vi "Transmit_Log_File_FGV.vi"(7 "Session name":string, 8 "error in (no error)":errorcluster, 9 "Command":enum16{"Initialize", "Update", "Stop"}(ring), 10 "Time (ms)":u32, 11 "Processed bytes":u8[](array[numeric])) -> (0 "error out":errorcluster, 3 "Receive Log File Path":path)   [LabVIEW 2017]
uses:
  <vilib>/Utility/file.llb/Write Delimited Spreadsheet (string).vi
  <vilib>/Utility/file.llb/Write Delimited Spreadsheet (I64).vi
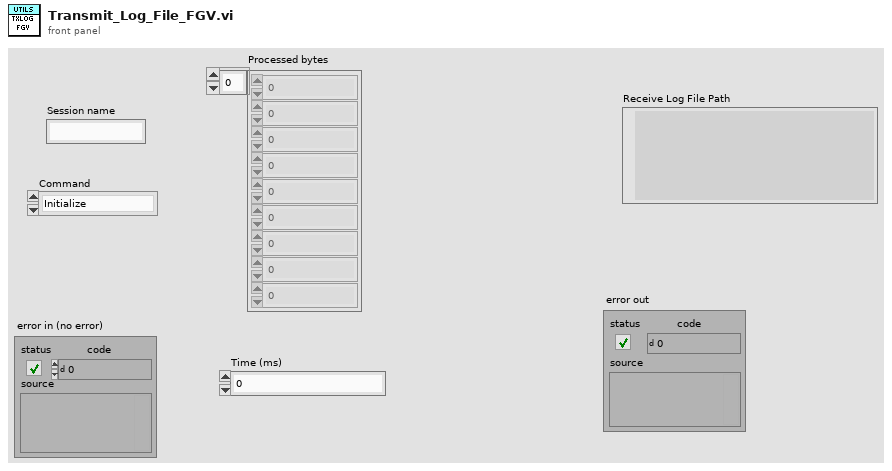
[diagram p1: front panel]
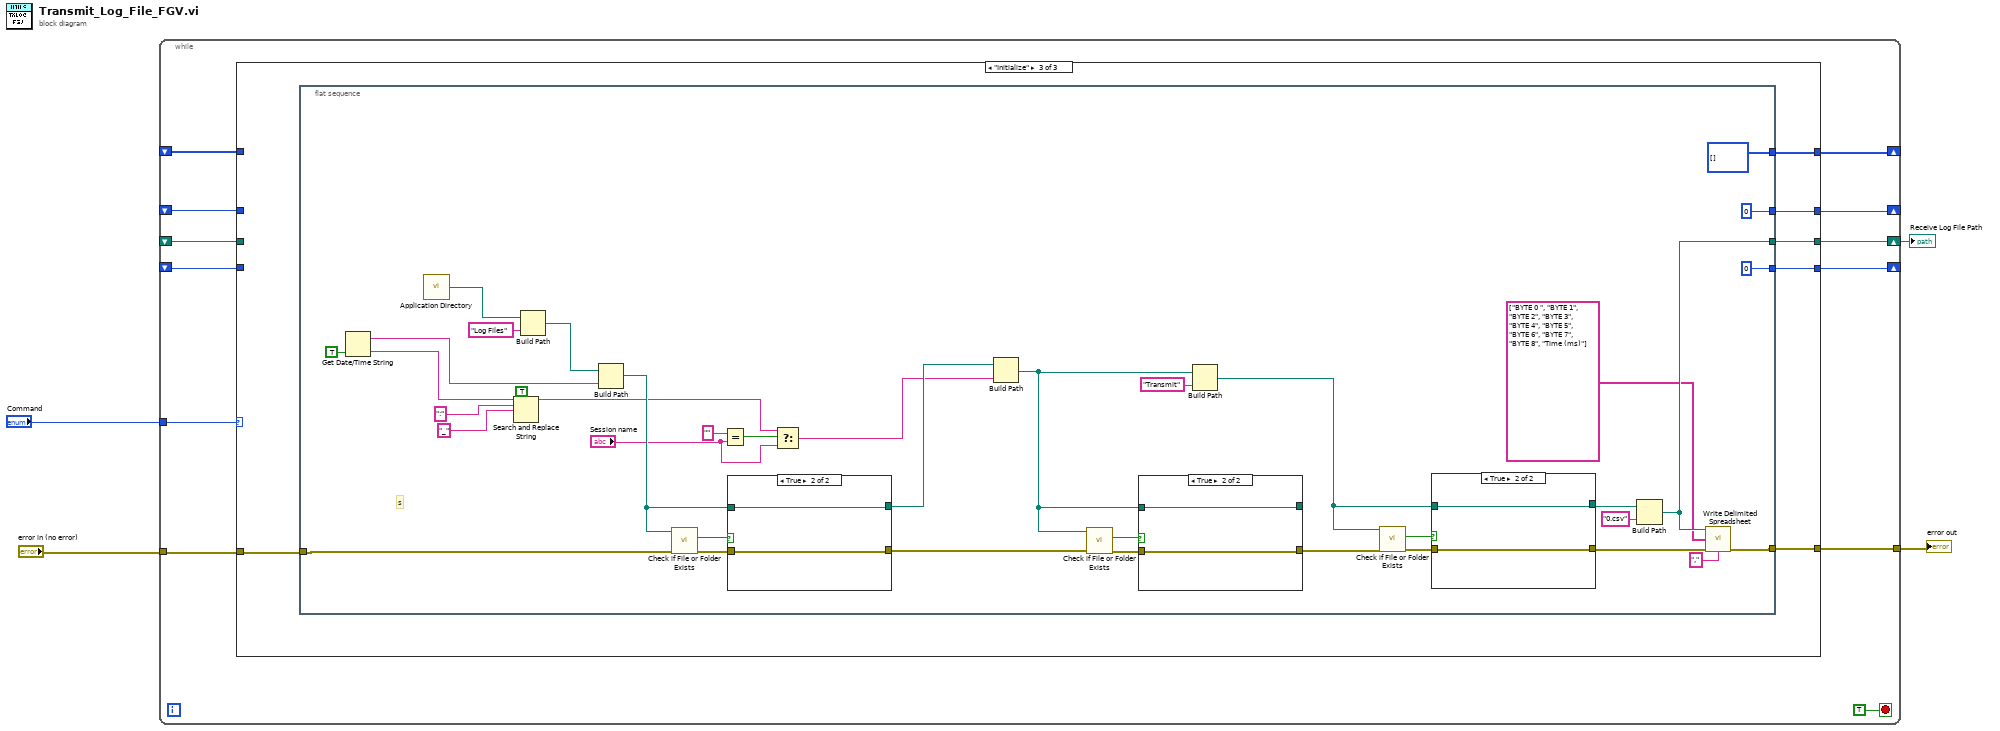
[diagram p0: block diagram]
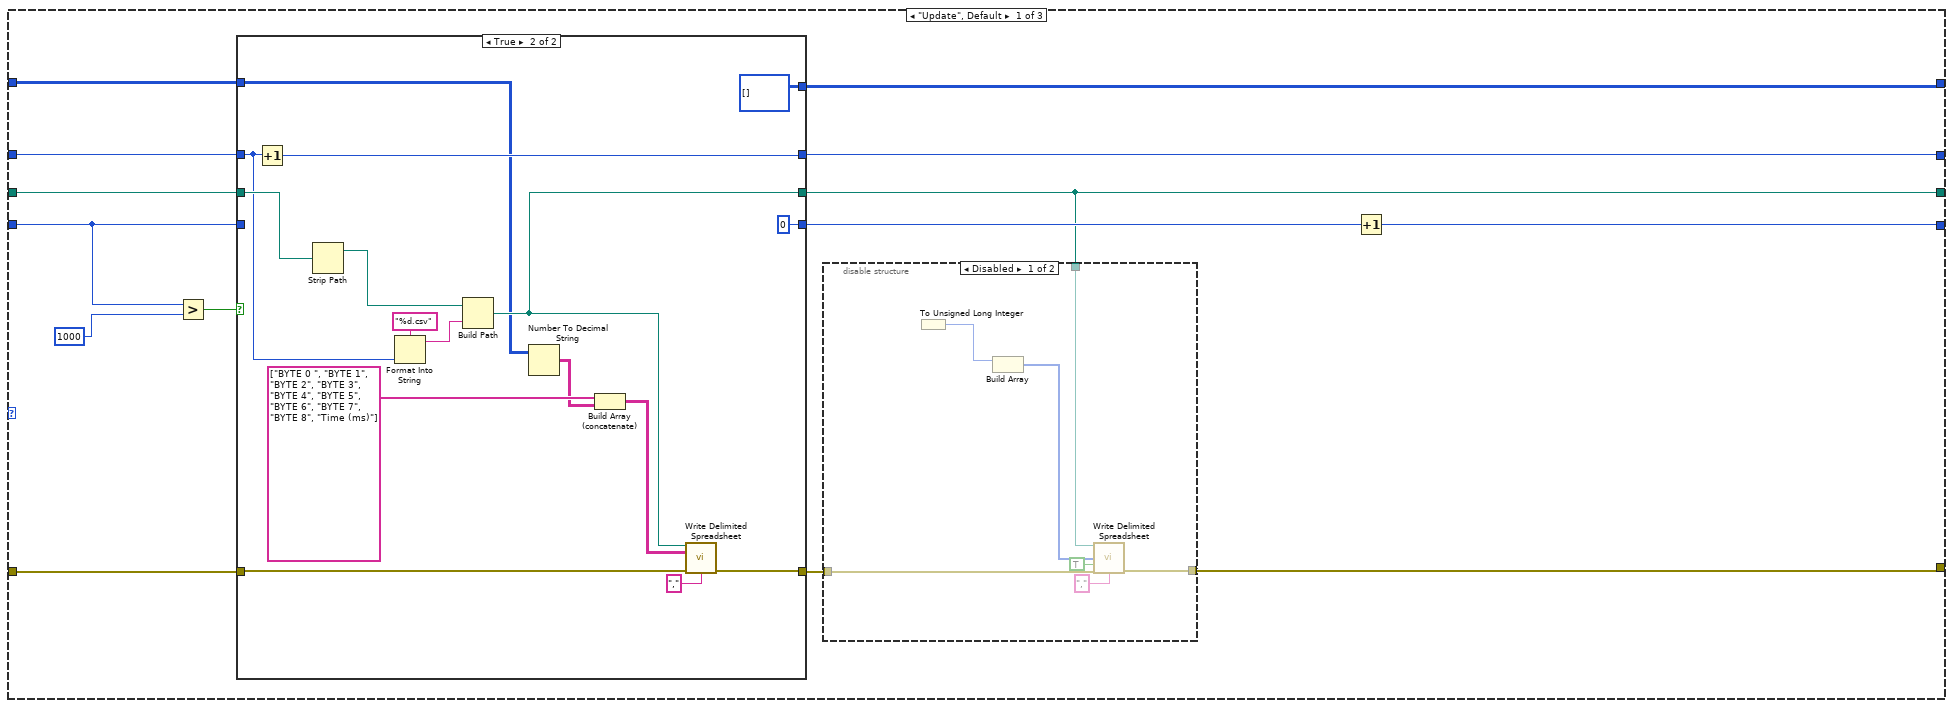
[diagram p2: hidden frame]
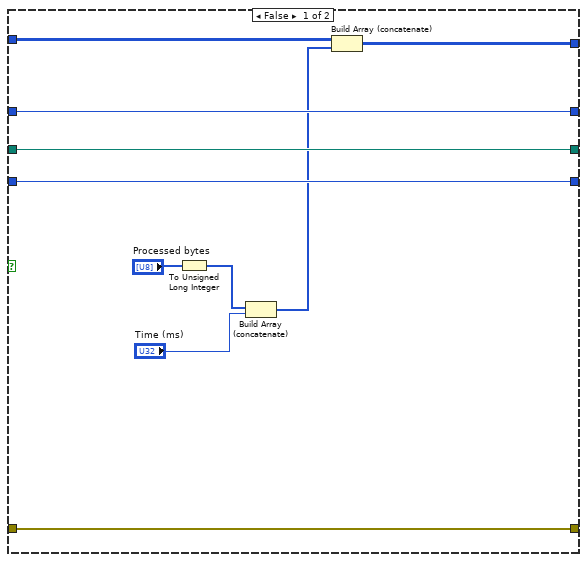
[diagram p4: hidden frame]
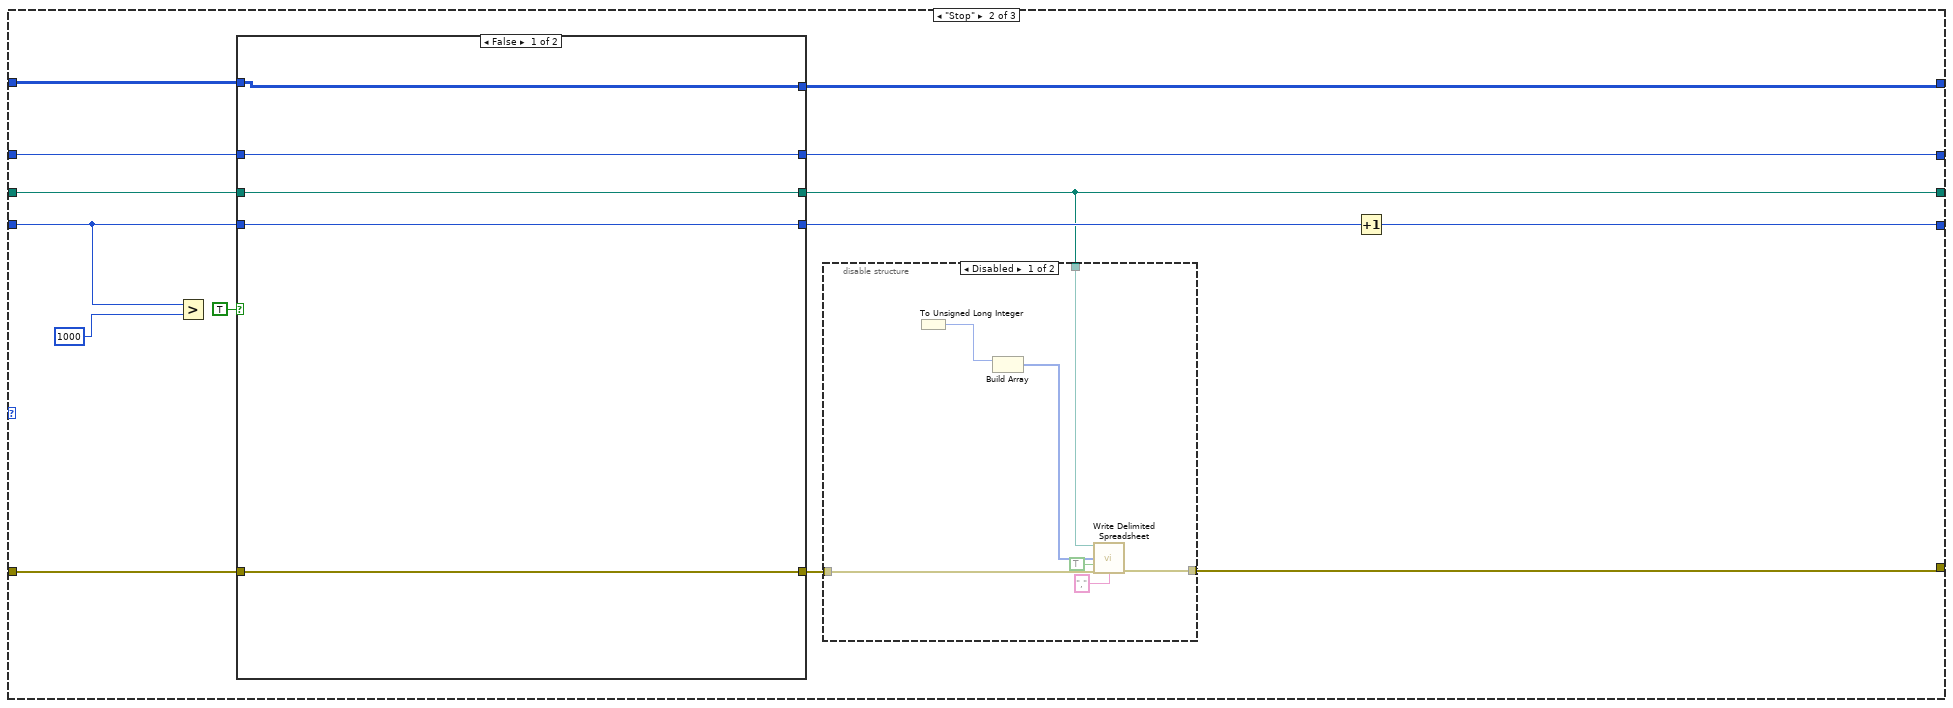
[diagram p5: hidden frame]
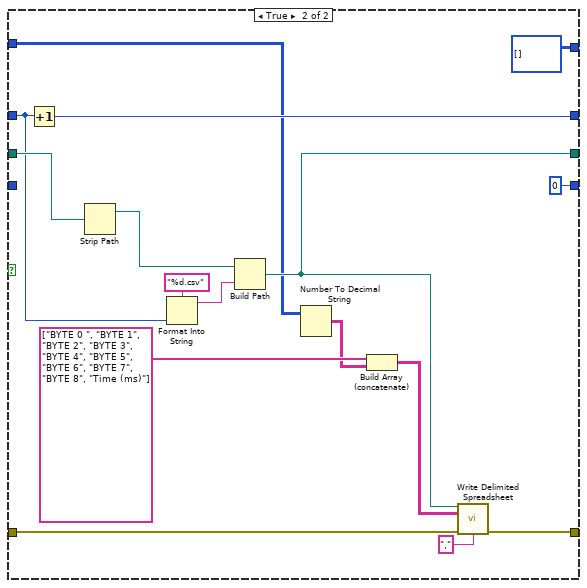
[diagram p7: hidden frame]
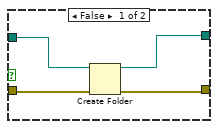
[diagram p8: hidden frame]
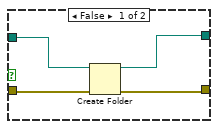
[diagram p9: hidden frame]
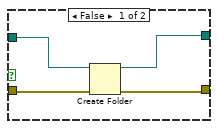
[diagram p10: hidden frame]
diagram:
  n1 = while {
    tunnel: "error in (no error)" -> [w16]
    tunnel: "Command" -> [w15]
    tunnel: [w13] -> w2
    shift-right: [w12] -> w3
    shift-left: _ -> [w9]
    shift-right: [w11] -> _
    shift-left: _ -> [w10]
    shift-right: [w8] -> _
    shift-left: _ -> [w7]
    shift-right: [w6] -> _
    shift-left: _ -> [w5]
    stop <- TRUE stop-if-true
    n2 = case shown="\"Initialize\"" w15 {
      tunnel: w16 -> [w30 w80 w117]
      tunnel: [w20 w71 w116] -> w13
      tunnel: [w21 w72 w115] -> w12
      tunnel: [w19 w70 w114] -> w11
      tunnel: w10 -> [w24 w75 _]
      tunnel: w9 -> [w27 w78 _]
      tunnel: [w25 w76 w113] -> w8
      tunnel: w7 -> [w26 w77 _]
      tunnel: [w17 w68 w112] -> w6
      tunnel: w5 -> [w18 w69 _]
      frame "Update", Default {
        n3 = Greater?(x=w24, y=1000) -> (0:w29:bool)
        n4 = case shown="True" w29 {
          tunnel: w30 -> [w49 w61]
          tunnel: [w49 w59] -> w22
          tunnel: w27 -> [w50 w66]
          tunnel: [w50 w58] -> w21
          tunnel: w26 -> [w48 w55]
          tunnel: [w48 w63] -> w25
          tunnel: w24 -> [w47 _]
          tunnel: [w47 0] -> w23
          tunnel: w18 -> [w43 w54]
          tunnel: [w41 u32[][] []] -> w17
          frame False {
            n5 = To Unsigned Long Integer(number="Processed bytes") -> (unsigned 32bit integer=w45:u32[])
            n6 = Build Array (concatenate)(w45, "Time (ms)") -> (w42:u32[])
            n7 = Build Array (concatenate)(w43, w42) -> (w41:u32[][])
          }
          frame True {
            n8 = Increment(x=w55) -> (x+1=w63:i32)
            n9 = Strip Path(path=w66) -> (stripped path=w65:path)  [unwired: 1 out]
            n10 = Format Into String(format string="%d.csv", w55) -> (resulting string=w62:string)  [unwired: 2 in, 1 out]
            n11 = Build Path(base path=w65, name or relative path=w62) -> (appended path=w58:path)
            n12 = Number To Decimal String(number=w54) -> (decimal integer string=w52:string[][])  [unwired: 1 in]
            n13 = Build Array (concatenate)(string[] ["BYTE 0 ", "BYTE 1", "BYTE 2", "BYTE 3", "BYTE 4", "BYTE 5", "BYTE 6", "BYTE 7", "BYTE 8", "Time (ms)"], w52) -> (w51:string[][])
            n14 = call-poly <vilib>:"Write Delimited Spreadsheet.vi"("file path (dialog if empty)"=w58, "2D data"=w51, "error in (no error)"=w61, "delimiter (\\t)"="," ("delimiter (\\t)")) -> ("error out"=w59:errorcluster)  [unwired: 10 in, 1 out]
          }
        }
        n15 = disable-structure shown="Disabled" {
          disable-tunnel: w22 -> [w39 w40]
          disable-tunnel: w21 -> [w38 _]
          disable-tunnel: [w35 w40] -> w20
          frame Disabled {
            n16 = To Unsigned Long Integer() -> (number=w34:u32, unsigned 32bit integer=w33:u32)
            n17 = Build Array(w33) -> (w31:u32[], w32:u32)
            n18 = call-poly <vilib>:"Write Delimited Spreadsheet.vi"("file path (dialog if empty)"=w38, "1D data"=w31, "append to file? (new file:F)"=TRUE, "error in (no error)"=w39, "delimiter (\\t)"="," ("delimiter (\\t)")) -> ("error out"=w35:errorcluster)  [unwired: 9 in, 1 out]
          }
          frame Enabled {
          }
        }
        n19 = Increment(x=w23) -> (x+1=w19:i32)
      }
      frame "Stop" {
        n20 = Greater?(x=w75, y=1000) -> ()  [unwired: 1 out]
        n21 = case shown="False" TRUE {
          tunnel: w80 -> [w94 w106]
          tunnel: [w94 w104] -> w73
          tunnel: w78 -> [w95 w111]
          tunnel: [w95 w103] -> w72
          tunnel: w77 -> [w93 w100]
          tunnel: [w93 w108] -> w76
          tunnel: w75 -> [w92 _]
          tunnel: [w92 0] -> w74
          tunnel: w69 -> [w91 w99]
          tunnel: [w91 u32[][] []] -> w68
          frame False {
          }
          frame True {
            n22 = Increment(x=w100) -> (x+1=w108:i32)
            n23 = Strip Path(path=w111) -> (stripped path=w110:path)  [unwired: 1 out]
            n24 = Format Into String(format string="%d.csv", w100) -> (resulting string=w107:string)  [unwired: 2 in, 1 out]
            n25 = Build Path(base path=w110, name or relative path=w107) -> (appended path=w103:path)
            n26 = Number To Decimal String(number=w99) -> (decimal integer string=w97:string[][])  [unwired: 1 in]
            n27 = Build Array (concatenate)(string[] ["BYTE 0 ", "BYTE 1", "BYTE 2", "BYTE 3", "BYTE 4", "BYTE 5", "BYTE 6", "BYTE 7", "BYTE 8", "Time (ms)"], w97) -> (w96:string[][])
            n28 = call-poly <vilib>:"Write Delimited Spreadsheet.vi"("file path (dialog if empty)"=w103, "2D data"=w96, "error in (no error)"=w106, "delimiter (\\t)"="," ("delimiter (\\t)")) -> ("error out"=w104:errorcluster)  [unwired: 10 in, 1 out]
          }
        }
        n29 = disable-structure shown="Disabled" {
          disable-tunnel: w73 -> [w89 w90]
          disable-tunnel: w72 -> [w88 _]
          disable-tunnel: [w85 w90] -> w71
          frame Disabled {
            n30 = To Unsigned Long Integer() -> (number=w84:u32, unsigned 32bit integer=w83:u32)
            n31 = Build Array(w83) -> (w81:u32[], w82:u32)
            n32 = call-poly <vilib>:"Write Delimited Spreadsheet.vi"("file path (dialog if empty)"=w88, "1D data"=w81, "append to file? (new file:F)"=TRUE, "error in (no error)"=w89, "delimiter (\\t)"="," ("delimiter (\\t)")) -> ("error out"=w85:errorcluster)  [unwired: 9 in, 1 out]
          }
          frame Enabled {
          }
        }
        n33 = Increment(x=w74) -> (x+1=w70:i32)
      }
      frame "Initialize" {
        n34 = flat-sequence {
          tunnel: w117 -> [w150]
          tunnel: [w127] -> w116
          tunnel: [w129] -> w115
          tunnel: [0] -> w114
          tunnel: [0] -> w113
          tunnel: [u32[][] []] -> w112
          frame #0 {
            # "s"
            n35 = Get Date/Time String(want seconds? (F)=TRUE) -> (date string=w151:string, time string=w145:string)  [unwired: 2 in]
            n36 = call <vilib>:"Application Directory.vi"() -> ("Application Directory"=w154:path)
            n37 = Search and Replace String(replace all?=TRUE ("replace all? (F)"), input string=w145, search string=":", replace string="_" ("replace string (\"\")")) -> (result string=w120:string)  [unwired: 4 in, 3 out]
            n38 = Build Path(base path=w154, name or relative path="Log Files") -> (appended path=w152:path)
            n39 = Build Path(base path=w152, name or relative path=w151) -> (appended path=w147:path)
            n40 = call <vilib>:"Check if File or Folder Exists.vi"("error in (no error)"=w150, "path"=w147) -> ("error out"=w148:errorcluster, "file or folder exists?"=w149:bool)  [unwired: 7 in, 1 out]
            n41 = Equal?(x="", y="Session name") -> (x = y?=w122:bool)
            n42 = case shown="True" w149 {
              tunnel: w148 -> [w171 w173]
              tunnel: [w169 w173] -> w139
              tunnel: w147 -> [w170 w172]
              tunnel: [w168 w172] -> w146
              frame False {
                n43 = Create Folder(path (use dialog)=w170, error in=w171) -> (created path=w168:path, error out=w169:errorcluster)  [unwired: 1 in, 1 out]
              }
              frame True {
              }
            }
            n44 = Select(t=w120, s=w122, f="Session name") -> (s? t:f=w119:string)
            n45 = Build Path(base path=w146, name or relative path=w119) -> (appended path=w138:path)
            n46 = call <vilib>:"Check if File or Folder Exists.vi"("error in (no error)"=w139, "path"=w138) -> ("error out"=w140:errorcluster, "file or folder exists?"=w141:bool)  [unwired: 7 in, 1 out]
            n47 = case shown="True" w141 {
              tunnel: w140 -> [w165 w167]
              tunnel: [w163 w167] -> w134
              tunnel: w138 -> [w164 w166]
              tunnel: [w162 w166] -> _
              frame False {
                n48 = Create Folder(path (use dialog)=w164, error in=w165) -> (created path=w162:path, error out=w163:errorcluster)  [unwired: 1 in, 1 out]
              }
              frame True {
              }
            }
            n49 = Build Path(base path=w138, name or relative path="Transmit") -> (appended path=w133:path)
            n50 = call <vilib>:"Check if File or Folder Exists.vi"("error in (no error)"=w134, "path"=w133) -> ("error out"=w135:errorcluster, "file or folder exists?"=w136:bool)  [unwired: 7 in, 1 out]
            n51 = case shown="True" w136 {
              tunnel: w135 -> [w159 w161]
              tunnel: [w157 w161] -> w132
              tunnel: w133 -> [w158 w160]
              tunnel: [w156 w160] -> w131
              frame False {
                n52 = Create Folder(path (use dialog)=w158, error in=w159) -> (created path=w156:path, error out=w157:errorcluster)  [unwired: 1 in, 1 out]
              }
              frame True {
              }
            }
            n53 = Build Path(base path=w131, name or relative path="0.csv") -> (appended path=w129:path)
            n54 = call-poly <vilib>:"Write Delimited Spreadsheet.vi"("file path (dialog if empty)"=w129, "1D data"=string[] ["BYTE 0 ", "BYTE 1", "BYTE 2", "BYTE 3", "BYTE 4", "BYTE 5", "BYTE 6", "BYTE 7", "BYTE 8", "Time (ms)"], "error in (no error)"=w132, "delimiter (\\t)"="," ("delimiter (\\t)")) -> ("error out"=w127:errorcluster)  [unwired: 10 in, 1 out]
          }
        }
      }
    }
  }
  "error out" <- w2
  "Receive Log File Path" <- w3
